vi "Initial Recipe.vi"(8 "error in (no error)":errorcluster, 11 "MASTER in":refnum<class "MASTER.lvclass">) -> (0 "error out":errorcluster, 3 "MASTER out":refnum<class "MASTER.lvclass">)   [LabVIEW 2014, in "Files Library.lvlib" / "MASTER.lvclass"]
uses:
  MASTER/MASTER.lvclass
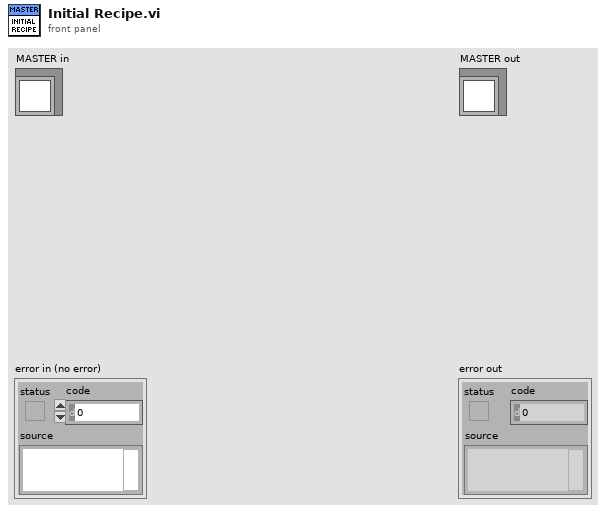
[diagram p1: front panel]
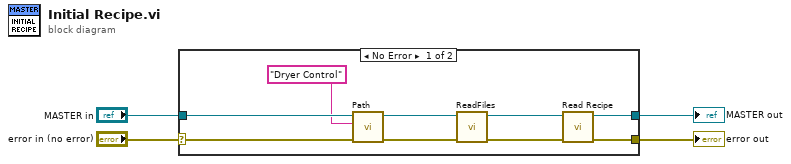
[diagram p0: block diagram]
diagram:
  n1 = case shown="No Error" "error in (no error)" {
    selector: "error in (no error)" -> [w13 w15]
    tunnel: [w5 w15] -> w3
    tunnel: [w6 w14] -> w1
    tunnel: "MASTER in" -> [w11 w14]
    frame No Error {
      n2 = call-dynamic "Path.vi"("error in (no error)"=w13, "pathname"="Dryer Control", "Master in"=w11) -> ("error out"=w12:errorcluster, "Master out"=w10:refnum<class "MASTER.lvclass">)  [unwired: 7 in]
      n3 = call-dynamic "ReadFiles.vi"("error in (no error)"=w12, "Master in"=w10) -> ("error out"=w7:errorcluster, "Master out"=w8:refnum<class "MASTER.lvclass">)  [unwired: 8 in]
      n4 = call-dynamic "Read Recipe.vi"("error in (no error)"=w7, "MASTER in"=w8) -> ("error out"=w5:errorcluster, "MASTER out"=w6:refnum<class "MASTER.lvclass">)  [unwired: 8 in]
    }
    frame Error {
    }
  }
  "error out" <- w3
  "MASTER out" <- w1
